vi "Remove Test Node.vi"(8 "error in (no error)":errorcluster, 11 "Test Node Model in":refnum<class "Test Node Model.lvclass">) -> (0 "error out":errorcluster, 3 "Test Node Model out":refnum<class "Test Node Model.lvclass">)   [LabVIEW 2013, in "Test Node Model.lvlib" / "Test Node Model.lvclass"]
uses:
  Test Node Model.lvclass
  Test Node Model.lvclass/Test Node Model.ctl
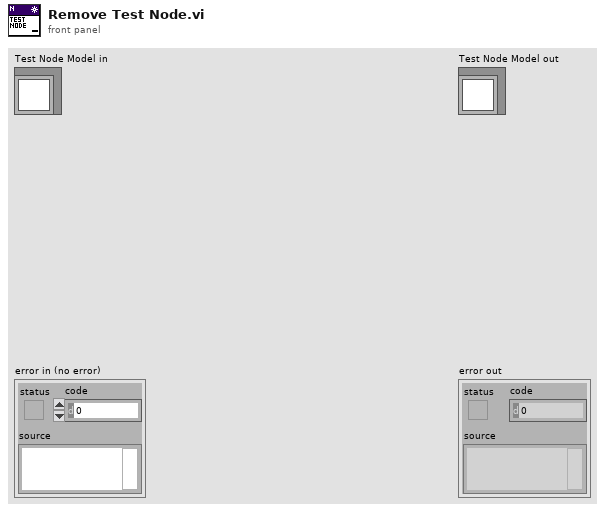
[diagram p1: front panel]
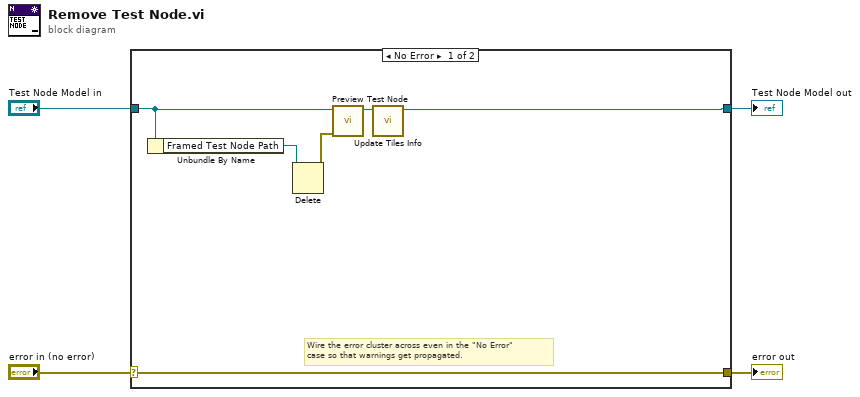
[diagram p0: block diagram]
diagram:
  n1 = case shown="No Error" "error in (no error)" {
    selector: "error in (no error)" -> [w10 w12]
    tunnel: [w10 w12] -> w3
    tunnel: [w5 w11] -> w1
    tunnel: "Test Node Model in" -> [w6 w11]
    frame No Error {
      # "Wire the error cluster across even in the \"No Error\"\ncase so that warnings get propagated."
      n2 = Unbundle By Name(w6) -> ("Framed Test Node Path"=w8:path)
      n3 = Delete(path (use dialog)=w8) -> (error out=w7:errorcluster)  [unwired: 4 in, 2 out]
      n4 = call "Preview Test Node.vi"("error in (no error)"=w7, "Test Node Model in"=w6) -> ("Test Node Model out"=w9:refnum<class "Test Node Model.lvclass">)  [unwired: 8 in, 1 out]
      n5 = call "Update Tiles Info.vi"("Test Node Model in"=w9) -> ("Test Node Model out"=w5:refnum<class "Test Node Model.lvclass">)  [unwired: 9 in, 1 out]
    }
    frame Error {
    }
  }
  "error out" <- w3
  "Test Node Model out" <- w1
